vi "SaveLoadTables.vi"(0 "Stop Program":refnum<vi>, 1 "Reactor Data":T1, 2 "Stop / Start Reactor X":refnum<vi>, 3 "Save Table Reactor X":refnum<vi>, 4 "Load Table Reactor X":refnum<vi>) -> ()   [LabVIEW 2021]
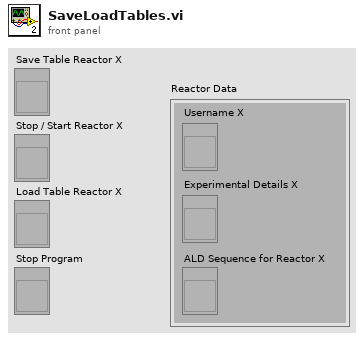
[diagram p1: front panel]
types:
  T1 = cluster{"ALD Sequence for Reactor X":refnum<vi>, "Username X":refnum<vi>, "Experimental Details X":refnum<vi>}
  T2 = cluster{"recipe":string[][], "username":string, "experimentalDetails":string}
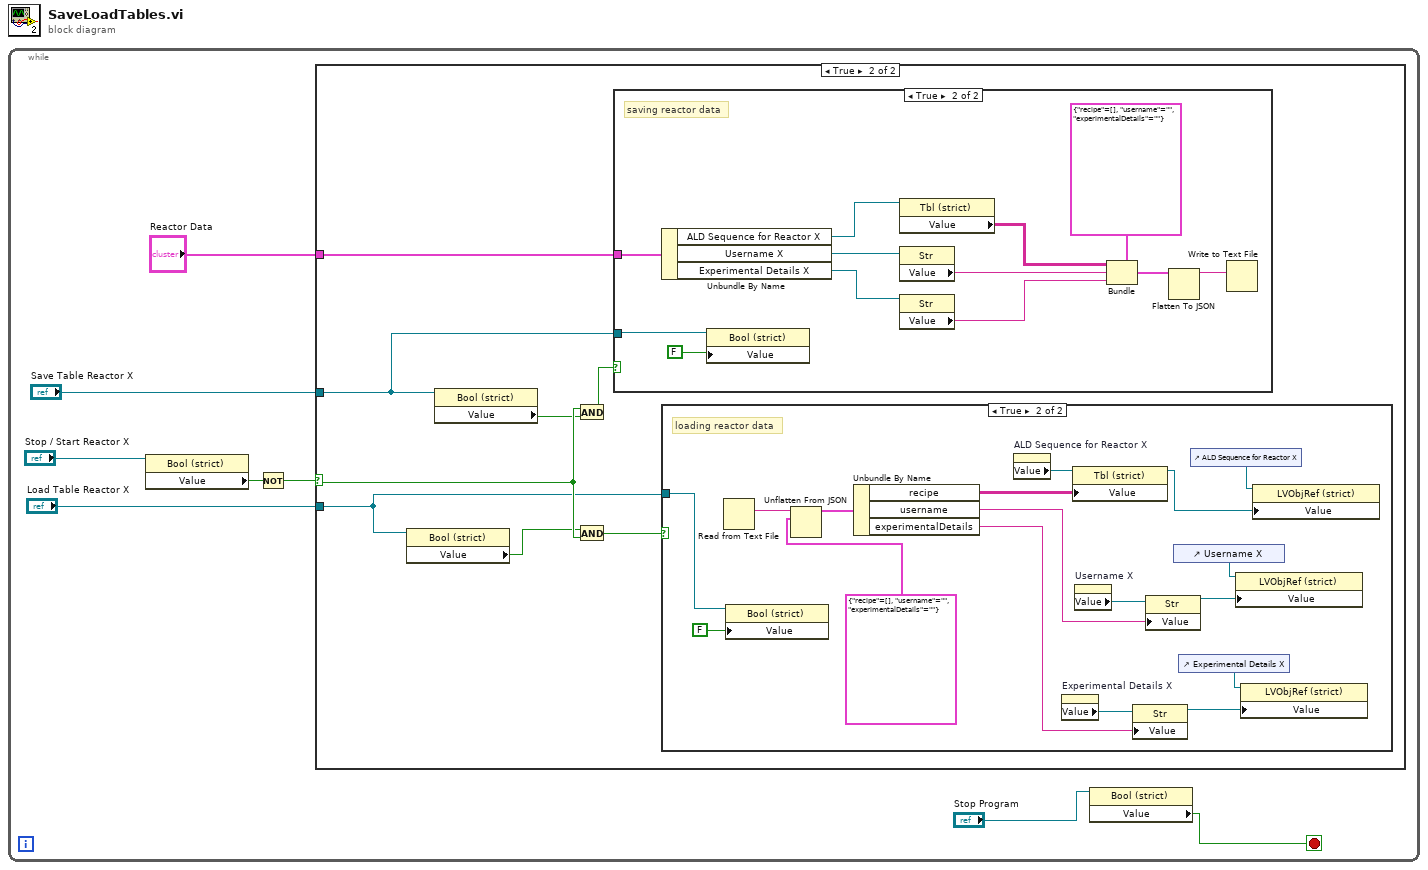
[diagram p0: block diagram]
diagram:
  n1 = while {
    stop <- w2 stop-if-true
    n2 = property class="Bool (strict)"(reference="Stop / Start Reactor X") -> ("Value"=w4:bool)  [unwired: 1 in, 2 out]
    n3 = Not(x=w4) -> (.not. x?=w5:bool)
    n4 = case shown="True" w5 {
      selector: w5 -> [_ w14]
      tunnel: "Load Table Reactor X" -> [_ w11]
      tunnel: "Save Table Reactor X" -> [_ w10]
      tunnel: "Reactor Data" -> [_ w9]
      frame False {
        # "Do nothing if a reactor is running."
      }
      frame True {
        n5 = property class="Bool (strict)"(reference=w11) -> ("Value"=w13:bool)  [unwired: 1 in, 2 out]
        n6 = property class="Bool (strict)"(reference=w10) -> ("Value"=w12:bool)  [unwired: 1 in, 2 out]
        n7 = And(x=w14, y=w12) -> (x .and. y?=w15:bool)
        n8 = And(x=w13, y=w14) -> (x .and. y?=w16:bool)
        n9 = case shown="True" w15 {
          tunnel: w10 -> [_ w26]
          tunnel: w9 -> [_ w20]
          frame False {
          }
          frame True {
            # "saving reactor data"
            n10 = Unbundle By Name(w20) -> ("ALD Sequence for Reactor X"=w19:refnum<vi>, "Username X"=w18:refnum<vi>, "Experimental Details X"=w17:refnum<vi>)
            n11 = property class="Bool (strict)"(reference=w26, "Value"=FALSE ("Save Table")) -> ()  [unwired: 1 in, 2 out]
            n12 = property class="Tbl (strict)"(reference=w19) -> ("Value"=w23:string[][])  [unwired: 1 in, 2 out]
            n13 = property class="Str"(reference=w18) -> ("Value"=w25:string)  [unwired: 1 in, 2 out]
            n14 = property class="Str"(reference=w17) -> ("Value"=w24:string)  [unwired: 1 in, 2 out]
            n15 = Bundle(cluster=T2 {"recipe"=[], "username"="", "experimentalDetails"=""}, "recipe"=w23, "username"=w25, "experimentalDetails"=w24) -> (w21:T2)
            n16 = Flatten To JSON(anything=w21) -> (JSON string=w27:string)  [unwired: 2 in, 1 out]
            n17 = Write to Text File(text=w27) -> ()  [unwired: 3 in, 3 out]
          }
        }
        n18 = case shown="True" w16 {
          tunnel: w11 -> [_ w44]
          frame False {
          }
          frame True {
            # "loading reactor data"
            n19 = Read from Text File() -> (text=w43:string)  [unwired: 4 in, 3 out]
            n20 = property class="Bool (strict)"(reference=w44, "Value"=FALSE ("Load Table")) -> ()  [unwired: 1 in, 2 out]
            n21 = Unflatten From JSON(JSON string=w43, type and defaults=T2 {"recipe"=[], "username"="", "experimentalDetails"=""} ("output cluster")) -> (value=w41:T2)  [unwired: 5 in, 1 out]
            n22 = Unbundle By Name(w41) -> ("recipe"=w40:string[][], "username"=w39:string, "experimentalDetails"=w38:string)
            n23 = property on="ALD Sequence for Reactor X" class="LVObjRef (strict)"() -> ("Value"=w29:refnum<vi>)  [unwired: 2 in, 2 out]
            n24 = property on="Experimental Details X" class="LVObjRef (strict)"() -> ("Value"=w30:refnum<vi>)  [unwired: 2 in, 2 out]
            n25 = property class="Tbl (strict)"(reference=w29, "Value"=w40) -> (reference out=w33:refnum<vi>)  [unwired: 1 in, 1 out]
            n26 = property on="Username X" class="LVObjRef (strict)"() -> ("Value"=w32:refnum<vi>)  [unwired: 2 in, 2 out]
            n27 = property class="Str"(reference=w30, "Value"=w38) -> (reference out=w35:refnum<vi>)  [unwired: 1 in, 1 out]
            n28 = property class="Str"(reference=w32, "Value"=w39) -> (reference out=w31:refnum<vi>)  [unwired: 1 in, 1 out]
            n29 = control-ref of="Username X"() -> (w37:refnum<vi>)
            n30 = control-ref of="Experimental Details X"() -> (w36:refnum<vi>)
            n31 = control-ref of="ALD Sequence for Reactor X"() -> (w34:refnum<vi>)
            n32 = property class="LVObjRef (strict)"(reference=w37, "Value"=w31) -> ()  [unwired: 1 in, 2 out]
            n33 = property class="LVObjRef (strict)"(reference=w36, "Value"=w35) -> ()  [unwired: 1 in, 2 out]
            n34 = property class="LVObjRef (strict)"(reference=w34, "Value"=w33) -> ()  [unwired: 1 in, 2 out]
          }
        }
      }
    }
    n35 = property class="Bool (strict)"(reference="Stop Program") -> ("Value"=w2:bool)  [unwired: 1 in, 2 out]
  }
